vi "Config Status.vi"(0 "Status report":T1(ring), 11 "error in (no error)":errorcluster) -> (15 "error out":errorcluster)   [LabVIEW 2024, in "GRBL 1.1.lvlib"]
doc: "Alters data included in status reports."
uses:
  GRBL 1.1.lvlib
panel:
  out "Data read":string
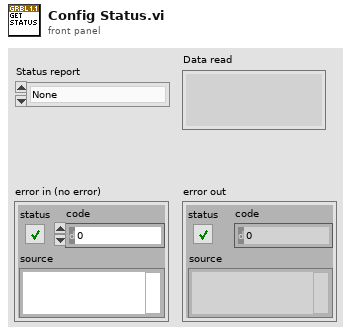
[diagram p1: front panel]
types:
  T1 = enum16{"None", "Machine position", "Work position", "Planner buffer", "RX Buffer", "Limit Pins"}
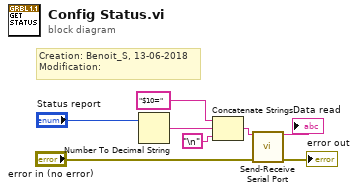
[diagram p0: block diagram]
diagram:
  # "Creation: Benoit_S, 13-06-2018\nModification:"
  n1 = Number To Decimal String(number="Status report") -> (decimal integer string=w3:string)  [unwired: 1 in]
  n2 = Concatenate Strings("$10=", w3, "\n") -> (w5:string)
  n3 = call "Send-Receive Serial Port.vi"("Data to write"=w5, "error in (no error)"="error in (no error)") -> ("Data read"=→"Data read":string, "error out"=→"error out":errorcluster)  [unwired: 12 in]
